vi "CRYProbe Curve.vi"() -> ()   [LabVIEW 2013]
panel:
  out "Source Step":string caption="源步骤"
  in  "Name":string
  in  "Update?":bool
  in  "Close?":bool
  in  "Number":i32
  out "Y unit":string caption="Y轴单位"
  out "X unit":string caption="X轴单位"
  out "End":dbl caption="结束" format="%#_6p"
  out "Start":dbl caption="开始" format="%#_6p"
  out "XY Graph":cluster{"XY Graph":cluster{dbl, dbl}[]}[](graph)
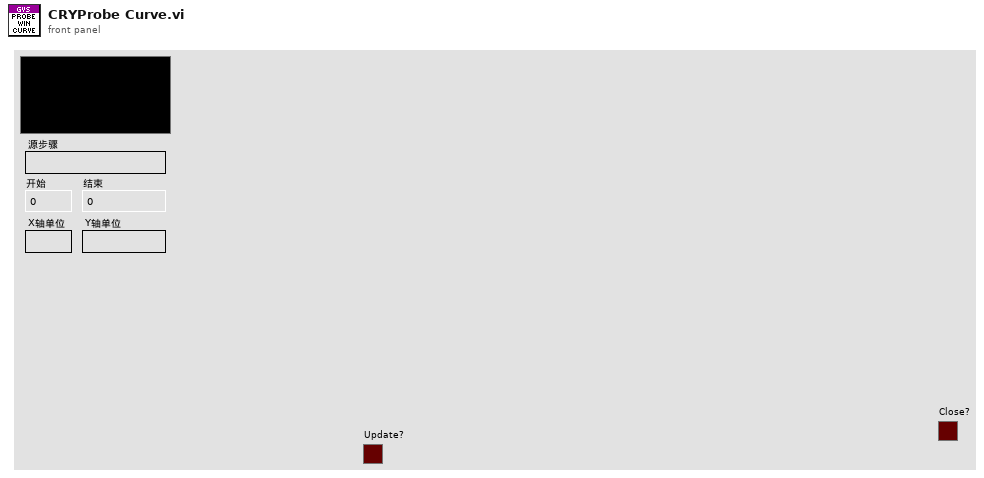
[diagram p1: front panel]
types:
  T1 = typedef "CRYData Cluster.ctl" = cluster{"Name":string, "Curve":cluster{"x":dbl, "y":dbl, "z":dbl}[], "X data":u16, "Y data":u16, "Z data":u16, "X axis":u16, "Y axis":u16, "Z axis":u16, "X unit":string, "Y unit":string, "Z unit":string, "X dB ref":dbl, "Y dB ref":dbl, "Z dB ref":dbl, "single val":bool, "protected":bool, "display X":bool, "display Y":bool, "display Z":bool, "Test Info":string, "Step No.":i32, "Plot Settings":cluster{"Color":u32, "Interpolation":u8, "Point Style":u8, "Line Style":u8, "Point Color":u32, "Line Width":u8, "Bar Plot Style":u8, "Fill To":i16}, "AutoProtect":bool}
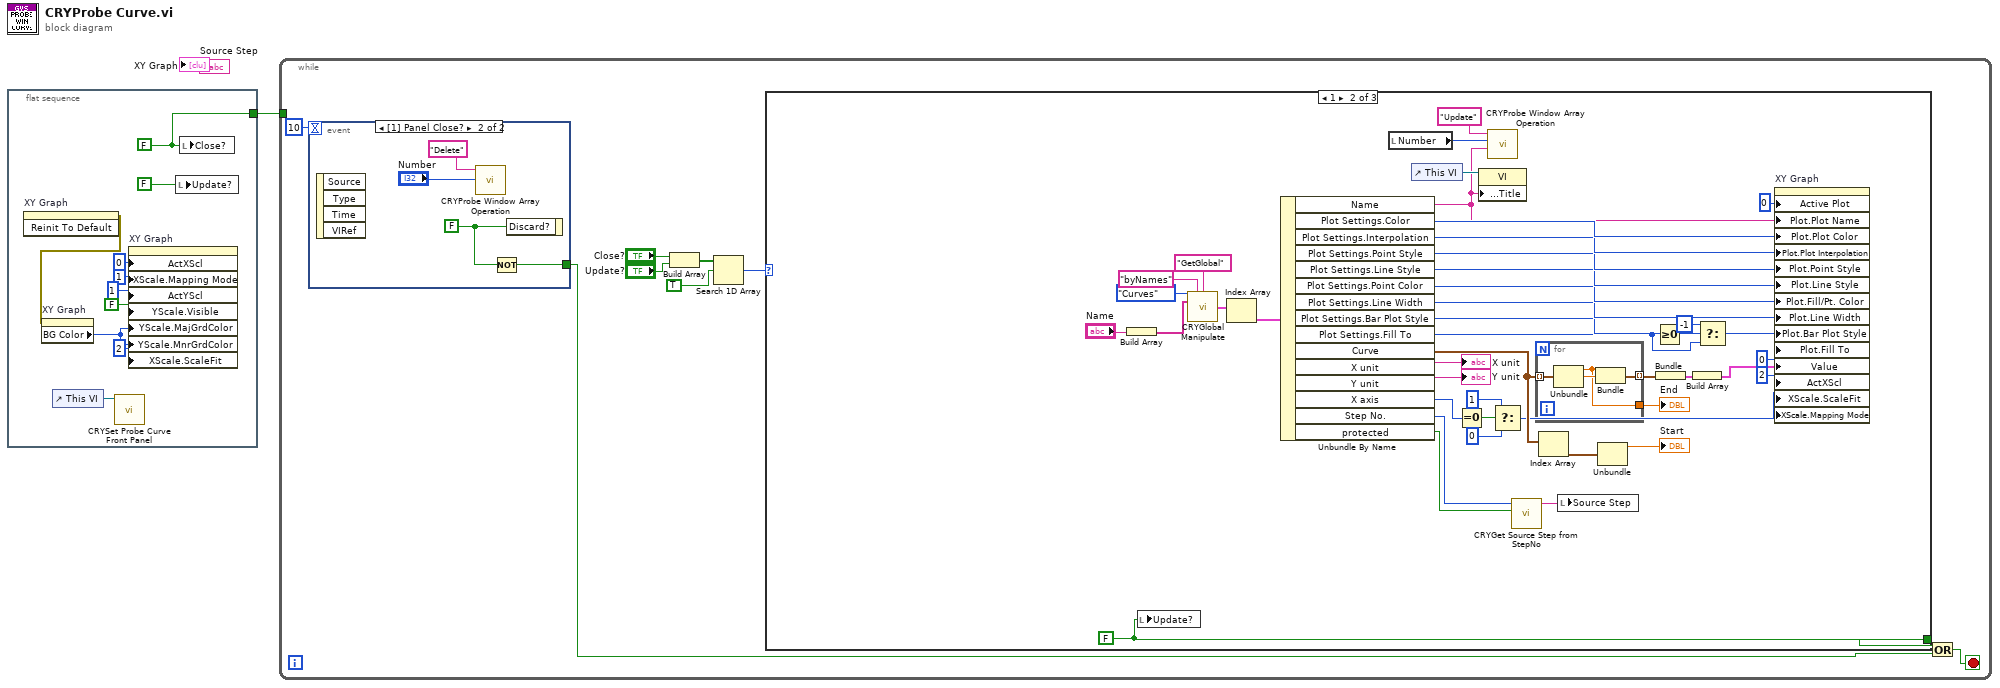
[diagram p0: block diagram]
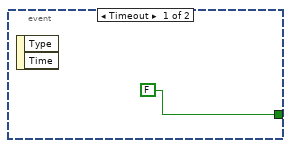
[diagram p2: hidden frame]
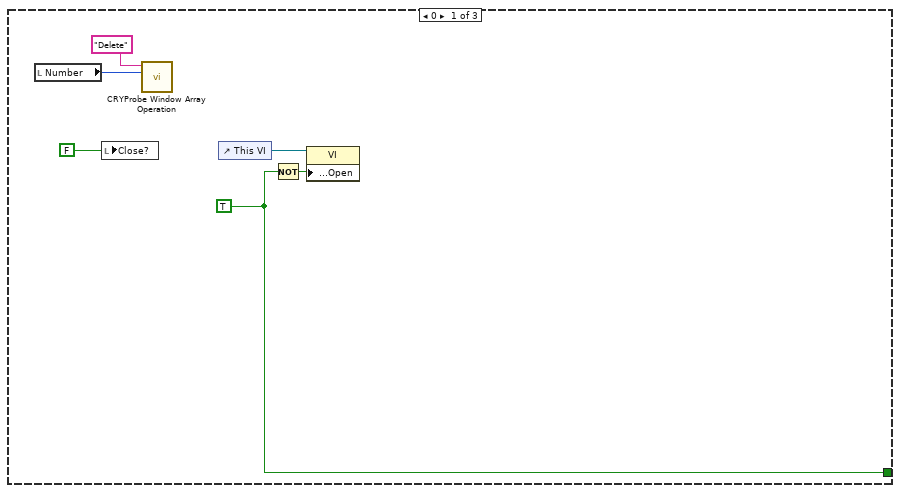
[diagram p3: hidden frame]
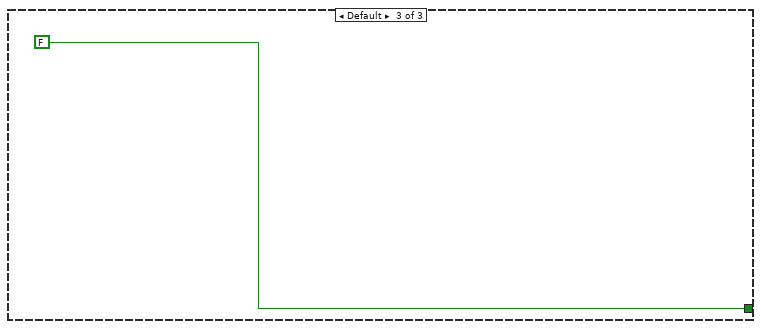
[diagram p4: hidden frame]
diagram:
  n1 = flat-sequence {
    tunnel: [w10] -> w1
    frame #0 {
      w10 = FALSE ("Close?")
      n2 = invoke on="XY Graph" class="XYGraph (strict)" method="Reinit To Default"() -> (error out=w3:errorcluster)  [unwired: 3 in, 2 out]
      n3 = property on="XY Graph" class="XYGraph (strict)"(error in=w3) -> ("BG Color"=w6:u32)  [unwired: 1 in, 2 out]
      n4 = control-ref of="This VI"() -> (w2:refnum<vi>)
      n5 = call "CRYSet Probe Curve Front Panel.vi"("Vi Ref"=w2) -> ()  [unwired: 11 in]
      n6 = property on="XY Graph" class="XYGraph (strict)"("ActXScl"=0 ("Active X Scale"), "XScale.Mapping Mode"=u8 1 ("X Scale.Mapping Mode"), "ActYScl"=1 ("Active Y Scale"), "YScale.Visible"=FALSE ("Y Scale.Visible"), "YScale.MajGrdColor"=w6, "YScale.MnrGrdColor"=w6, "XScale.ScaleFit"=u8 2 ("X Scale.Scale Fit")) -> ()  [unwired: 2 in, 2 out]
      n7 = local write "Update?"(FALSE ("Close?")) -> ()
      n8 = local write "Close?"(w10) -> ()
    }
  }
  n9 = while {
    tunnel: w1 -> [_]
    stop <- w15 stop-if-true
    n10 = event shown="[1] Panel Close?" {
      selector: _ -> [_ _]
      dyn-events: _ -> [_ _]
      timeout: 10 -> [_ _]
      tunnel: [FALSE ("Discard?") w24] -> w12
      event Timeout {
        n11 = event-data() -> ()  [unwired: 3 out]
      }
      event Panel Close? {
        w25 = FALSE ("Discard?")
        n12 = event-data() -> ()  [unwired: 5 out]
        n13 = call "CRYProbe Window Array Operation.vi"("Number"="Number", "sAction"="Delete") -> ()  [unwired: 1 in, 9 out]
        n14 = Not(x=w25) -> (.not. x?=w24:bool)
        n15 = event-data("Discard?"=w25) -> ()  [unwired: 1 in, 1 out]
      }
    }
    n16 = Build Array("Close?", "Update?") -> (w18:bool[])
    n17 = Search 1D Array(1D array=w18, element=TRUE) -> (index of element=w19:i32)  [unwired: 1 out]
    n18 = case shown="1" w19 {
      tunnel: [w30 w74 FALSE ("Close?")] -> w16
      frame 0 {
        w30 = TRUE ("Discard?")
        n19 = local read "Number"() -> (w26:i32)
        n20 = local write "Close?"(FALSE ("Close?")) -> ()
        n21 = call "CRYProbe Window Array Operation.vi"("Number"=w26, "sAction"="Delete") -> ()  [unwired: 1 in, 9 out]
        n22 = control-ref of="This VI"() -> (w28:refnum<vi>)
        n23 = Not(x=w30) -> (.not. x?=w31:bool)
        n24 = property class="VI"(reference=w28, "Front Panel.Open"=w31) -> ()  [unwired: 1 in, 2 out]
      }
      frame 1 {
        w74 = FALSE ("Close?")
        n25 = Build Array("Name") -> (w32:string[])
        n26 = local write "Update?"(w74) -> ()
        n27 = call "CRYGlobal Manipulate.vi"("Type"=enum16{"Curves", "Values", "Results", "WFM"}."Curves" ("Type In"), "sOption"="byNames", "sAction"="GetGlobal", "sData"=w32) -> ("Curves Out"=w37:T1[])  [unwired: 5 in, 6 out]
        n28 = Index Array(array=w37) -> (element=w36:T1)  [unwired: 1 in]
        n29 = Unbundle By Name(w36) -> ("Name"=w54:string, "Plot Settings.Color"=w65:u32, "Plot Settings.Interpolation"=w51:u8, "Plot Settings.Point Style"=w50:u8, "Plot Settings.Line Style"=w49:u8, "Plot Settings.Point Color"=w48:u32, "Plot Settings.Line Width"=w47:u8, "Plot Settings.Bar Plot Style"=w46:u8, "Plot Settings.Fill To"=w42:i16, "Curve"=w70:cluster{"x":dbl, "y":dbl, "z":dbl}[], "X unit"=→"X unit":string, "Y unit"=→"Y unit":string, "X axis"=w55:u16, "Step No."=w41:i32, "protected"=w40:bool)
        n30 = local read "Number"() -> (w53:i32)
        n31 = control-ref of="This VI"() -> (w63:refnum<vi>)
        n32 = Equal To 0?(x=w55) -> (x = 0?=w57:bool)
        n33 = property class="VI"(reference=w63, "Front Panel.Title"=w54) -> ()  [unwired: 1 in, 2 out]
        n34 = call "CRYProbe Window Array Operation.vi"("Name"=w54, "Number"=w53, "sAction"="Update") -> ()  [unwired: 9 out]
        n35 = Select(t=u8 1, s=w57, f=u8 0) -> (s? t:f=w56:u8)
        n36 = call "CRYGet Source Step from StepNo.vi"("Protect?"=w40, "Step No."=w41) -> ("StepName"=w39:string)  [unwired: 9 in]
        n37 = for {
          tunnel: w70 -> [w77] mode=indexing
          tunnel: [w76] -> w67 mode=indexing
          tunnel: [w75] -> w73
          n38 = Unbundle(w77) -> ("x"=w75:dbl, "y"=w78:dbl)  [unwired: 1 out]
          n39 = Bundle("x"=w75, "y"=w78) -> (w76:cluster{"x":dbl, "y":dbl})  [unwired: 1 out]
        }
        "End" <- w73
        n40 = Index Array(array=w70) -> (element=w71:cluster{"x":dbl, "y":dbl, "z":dbl})  [unwired: 1 in]
        n41 = local write "Source Step"(w39) -> ()
        n42 = Unbundle(w71) -> ("x"=→"Start":dbl)  [unwired: 2 out]
        n43 = Greater Or Equal To 0?(x=w42) -> (x >= 0?=w43:bool)
        n44 = Bundle(w67) -> (w66:cluster{cluster{"x":dbl, "y":dbl}[]})  [unwired: 1 in]
        n45 = Build Array(w66) -> (w64:cluster{cluster{"x":dbl, "y":dbl}[]}[])
        n46 = Select(t=i16 -1 ("Fill To"), s=w43, f=w42) -> (s? t:f=w44:i16)
        n47 = property on="XY Graph" class="XYGraph (strict)"("Active Plot"=u32 0, "Plot.Plot Name"=w54, "Plot.Plot Color"=w65, "Plot.Plot Interpolation"=w51, "Plot.Point Style"=w50, "Plot.Line Style"=w49, "Plot.Fill/Pt. Color"=w48, "Plot.Line Width"=w47, "Plot.Bar Plot Style"=w46, "Plot.Fill To"=w44, "Value"=w64, "ActXScl"=0 ("Active X Scale"), "XScale.ScaleFit"=u8 2 ("X Scale.Scale Fit"), "XScale.Mapping Mode"=w56) -> ()  [unwired: 2 in, 2 out]
      }
      frame Default {
      }
    }
    n48 = Or(x=w16, y=w12) -> (x .or. y?=w15:bool)
  }
